vi "Init Actor.vi"() -> (2 "Actor":refnum<class "Actor.lvclass">)   [LabVIEW 2020, in "_Template.lvlib" / "Templates.lvlib" / "TEMPLATE jettl Actor.lvlib" / "TEMPLATE.lvlib"]
uses:
  TEMPLATE.lvlib
  jettl/jettl/Actor/Actor.lvclass
  TEMPLATE Actor/TEMPLATE Actor.lvlib
panel:
  # "This front panel should not be manipulated."
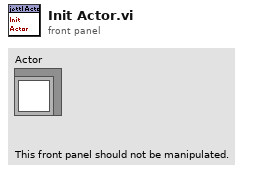
[diagram p1: front panel]
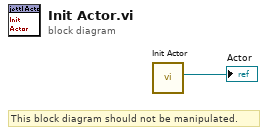
[diagram p0: block diagram]
diagram:
  # "This block diagram should not be manipulated."
  n1 = call "Init Actor.vi"() -> ("Actor"=→"Actor":refnum<class "Actor.lvclass">)  [unwired: 11 in]
